vi "Exercise 5.5.vi"() -> ()   [LabVIEW 2020]
panel:
  out "Gauge 6":dbl(knob) scale=0.0..10.0
  out "Gauge 5":dbl(knob) scale=0.0..10.0
  out "Gauge 4":dbl(knob) scale=0.0..10.0
  out "Gauge 3":dbl(knob) scale=0.0..10.0
  out "Gauge 2":dbl(knob) scale=0.0..10.0
  out "Gauge":dbl(knob) scale=0.0..10.0
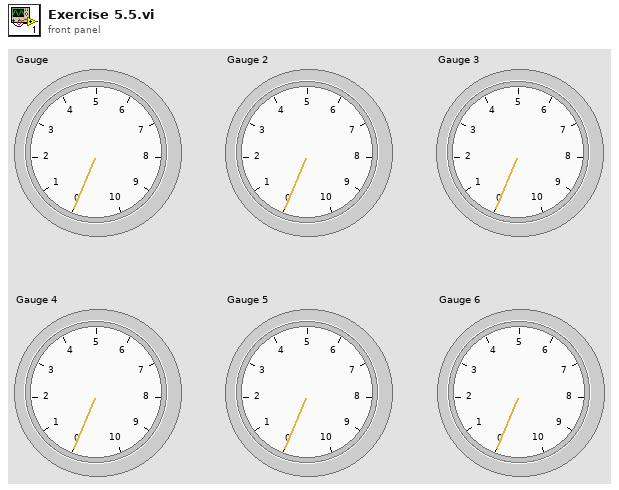
[diagram p1: front panel]
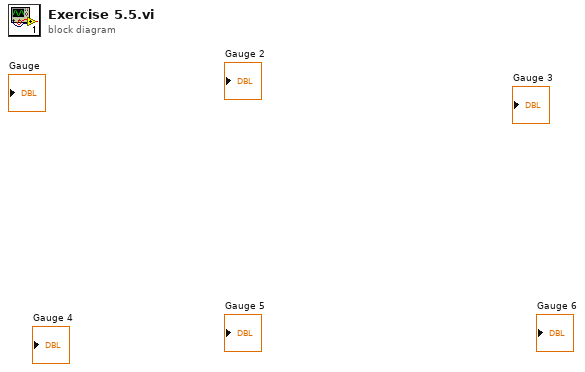
[diagram p0: block diagram]
diagram:
